vi "Unflatten.vi"(8 "error in (no error)":errorcluster, 11 "Wavelength in":refnum<class "Wavelength Triax 550.lvclass">) -> (0 "error out":errorcluster, 3 "Wavelength out":refnum<class "Wavelength Triax 550.lvclass">)   [LabVIEW 2017, in "Wavelength Triax 550.lvclass"]
uses:
  Wavelength Triax 550.lvclass
  Wavelength Triax 550.lvclass/Wavelength Triax 550.ctl
  Global/File Locations.vi
  Scanner/Scanner.lvclass
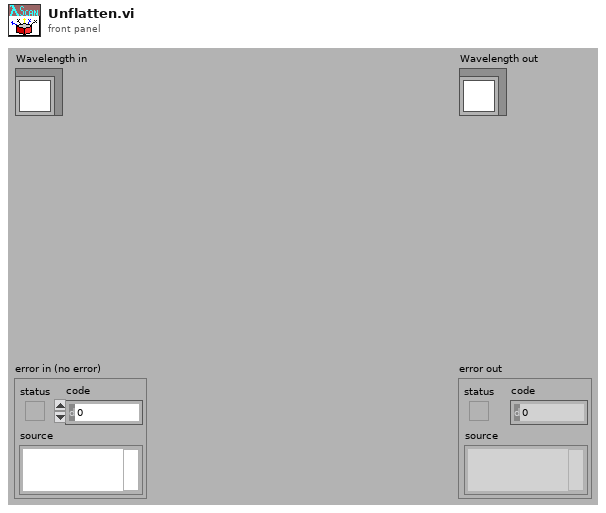
[diagram p1: front panel]
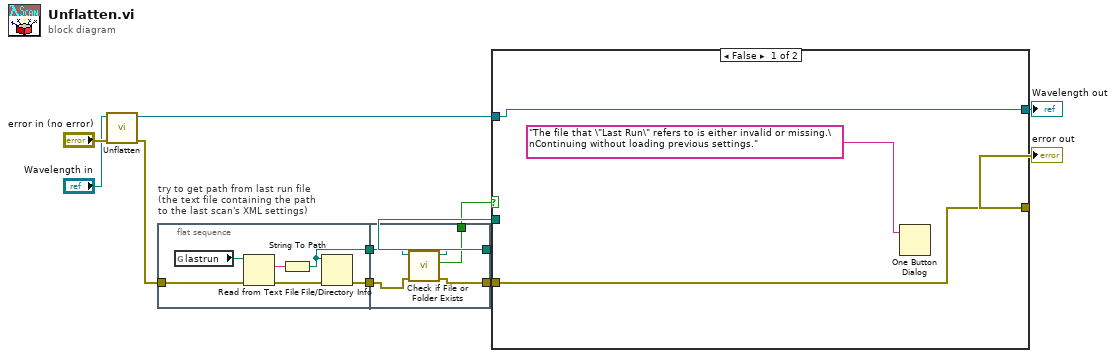
[diagram p0: block diagram]
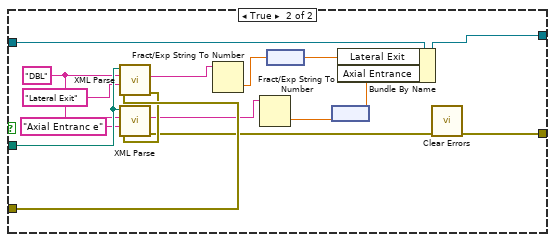
[diagram p2: hidden frame]
diagram:
  n1 = call-parent "Unflatten.vi"("error in (no error)"="error in (no error)", "Scanner in"="Wavelength in") -> ("error out"=w7:errorcluster, "Scanner out"=w11:refnum<class "Wavelength Triax 550.lvclass">)  [unwired: 8 in]
  n2 = flat-sequence "try to get path from last run file\n(the text file containing the path\nto the last scan's XML settings)" {
    tunnel: w7 -> [w12]
    tunnel: [w17] -> w3
    tunnel: [w13] -> w2
    tunnel: [w20] -> w5
    tunnel: [w21] -> w6
    tunnel: w3 -> [w22]
    tunnel: w2 -> [w19]
    tunnel: [w18] -> w1
    frame #0 {
      n3 = global read "File Locations.vi" "lastrun"() -> (w15:path)
      n4 = Read from Text File(file (use dialog)=w15, error in=w12) -> (text=w16:string, error out=w14:errorcluster)  [unwired: 4 out]
      n5 = String To Path(string=w16) -> (path=w17:path)
      n6 = File/Directory Info(path=w17, error in=w14) -> (error out=w13:errorcluster)  [unwired: 6 out]
    }
    frame #1 {
      n7 = call <vilib>:"Check if File or Folder Exists.vi"("error in (no error)"=w19, "path"=w22) -> ("error out"=w20:errorcluster, "file or folder exists?"=w18:bool, "dup path"=w21:path)  [unwired: 7 in]
    }
  }
  n8 = case shown="False" w1 {
    tunnel: w11 -> [w24 w41]
    tunnel: [w24 w40] -> w8
    tunnel: w6 -> [_ w39]
    tunnel: w5 -> [w25 w35]
    tunnel: [w25 w26] -> w4
    frame False {
      n9 = One Button Dialog(message="The file that \"Last Run\" refers to is either invalid or missing.\nContinuing without loading previous settings.") -> ()  [unwired: 1 in, 1 out]
    }
    frame True {
      w38 = "DBL"
      n10 = call "XML Parse.vi"("error in (no error)"=w35, "Name String"="Lateral Exit", "Type String"=w38, "Path"=w39) -> ("error out"=w34:errorcluster, "String Out"=w32:string)  [unwired: 6 in]
      n11 = call "XML Parse.vi"("error in (no error)"=w34, "Name String"="Axial Entranc e", "Type String"=w38, "Path"=w39) -> ("error out"=w33:errorcluster, "String Out"=w31:string)  [unwired: 6 in]
      n12 = Fract/Exp String To Number(string=w32) -> (number=w30:dbl)  [unwired: 3 in, 1 out]
      n13 = Fract/Exp String To Number(string=w31) -> (number=w29:dbl)  [unwired: 3 in, 1 out]
      n14 = node(w30) -> (w28:dbl[unit])
      n15 = node(w29) -> (w27:dbl[unit])
      n16 = Bundle By Name(cluster=w41, "Lateral Exit"=w28, "Axial Entrance"=w27) -> (w40:refnum<class "Wavelength Triax 550.lvclass">)
      n17 = call <vilib>:"Clear Errors.vi"("error in (no error)"=w33) -> ("error out"=w26:errorcluster)  [unwired: 5 in, 1 out]
    }
  }
  "error out" <- w4
  "Wavelength out" <- w8
